vi "NI_FPGA_PPG.id query.vi"(0 "i ref in":refnum<vi>, 3 "ms timeout (10000)":i32=10000, 5 "error in (no error)":errorcluster) -> (14 "i ref out":refnum<vi>, 16 "IDString":string, 17 "timed out":bool, 19 "error out":errorcluster)   [LabVIEW 2014, in "NI_FPGA_PPG.lvlib"]
doc: "Performs an ID query of the device."
uses:
  NI_FPGA_PPG.lvlib
  CS_Core/CSApplicationBaseClasses/DeviceBase/DeviceBase.lvlib
  instr.lib/NI-FPGA-PPG/host/instrumentDriver/NI-FPGA-PPG_Driver.lvlib
  CSlibraries/UtilityLib/UtilityLib.lvlib
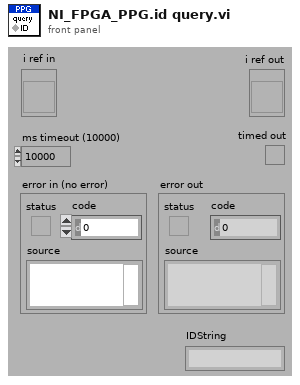
[diagram p1: front panel]
types:
  T1 = typedef "NI_FPGA_PPG.lvlib/NI_FPGA_PPG.i attribute.ctl" = cluster{"dim_service_id":cluster{"dim_actual_device_status":i32, "dim_event_data":i32, "dim_cmd_data":i32, "dim_cmd_data _description":i32, "dim_channel_description":i32}, "VISA":refnum<visa-resource-name>, "actual_device_status":i32, "event_data_id":i32, "pdc_enabled":bool, "pdc_timestamp":u32, "cmd_data_string":string, "cmd_data_size":i32, "cmd_data_description_string":string, "cmd_data_description_size":i32, "channel_description_string":string, "channel_description_size":i32}
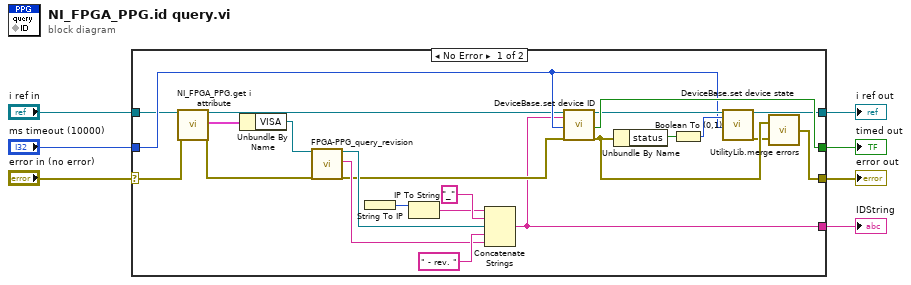
[diagram p0: block diagram]
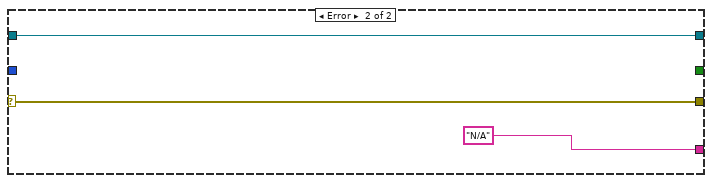
[diagram p2: hidden frame]
diagram:
  n1 = case shown="No Error" "error in (no error)" {
    selector: "error in (no error)" -> [w23 w32]
    tunnel: [w30 _] -> w7
    tunnel: [w26 w33] -> w6
    tunnel: "ms timeout (10000)" -> [w25 _]
    tunnel: "i ref in" -> [w24 w33]
    tunnel: [w10 w32] -> w2
    tunnel: [w11 "N/A"] -> w1
    frame No Error {
      n2 = call "NI_FPGA_PPG.get i attribute.vi"("i ref in"=w24, "error in (no error)"=w23) -> ("i ref out"=w22:refnum<vi>, "i attribute"=w21:T1, "error out"=w19:errorcluster)  [unwired: 15 in]
      n3 = Unbundle By Name(w21) -> ("VISA"=w20:refnum<visa-resource-name>)
      n4 = call "FPGA-PPG_query_revision.vi"("resource_in"=w20, "error in (no error)"=w19) -> ("resource_out"=w14:refnum<visa-resource-name>, "revision"=w13:string, "error out"=w12:errorcluster)  [unwired: 15 in]
      n5 = String To IP() -> (0:w16:u32)  [unwired: 1 in]
      n6 = IP To String(2:w16) -> (0:w17:string)  [unwired: 1 in]
      n7 = Concatenate Strings(w17, "_" ("string"), w14, " - rev. " ("string"), w13) -> (w11:string)
      n8 = call "DeviceBase.set device ID.vi"("i ref in"=w22, "deviceID"=w11, "ms timeout (10000)"=w25, "error in (no error)"=w12) -> ("i ref out"=w27:refnum<vi>, "timed out"=w30:bool, "error out"=w9:errorcluster)  [unwired: 13 in]
      n9 = Unbundle By Name(w9) -> ("status"=w29:bool)
      n10 = Boolean To (0,1)(Boolean=w29) -> (0, 1=w28:i16)
      n11 = call "DeviceBase.set device state.vi"("i ref in"=w27, "deviceState"=w28, "ms timeout (10000)"=w25) -> ("i ref out"=w26:refnum<vi>, "error out"=w8:errorcluster)  [unwired: 14 in, 1 out]
      n12 = call "UtilityLib.merge errors.vi"("error2 (no error)"=w8, "error1 (no error)"=w9) -> ("error out"=w10:errorcluster)
    }
    frame Error {
    }
  }
  "error out" <- w2
  "i ref out" <- w6
  "timed out" <- w7
  "IDString" <- w1
